vi "test Subset.vi"(8 "error in (no error)":errorcluster, 11 "TestCase in":refnum<class "Buffers Tests.lvclass">) -> (0 "error out":errorcluster, 3 "TestCase out":refnum<class "Buffers Tests.lvclass">)   [LabVIEW 2017, in "Buffers Tests.lvclass"]
uses:
  Buffers Tests.lvclass
  Buffers Tests.lvclass/Buffers Tests.ctl
  Classes/Buffers/Buffers.lvclass/Buffers.ctl
  <vilib>/NI/Memory Manager/Classes/Pointer/Pointer.lvclass/Pointer.ctl
  <vilib>/NI/Memory Manager/Classes/Pointer/Get Address.vi
  <vilib>/NI/Memory Manager/Classes/Pointer/Get Size.vi
  Classes/Buffer/Buffer.lvclass
  C:/Program Files (x86)/National Instruments/LabVIEW 2017/vi.lib/NI/Memory Manager/Classes/Pointer/Pointer.lvclass
  <vilib>/addons/_JKI Toolkits/VI Tester/TestCase.llb/TestCase.lvclass
  Classes/Buffers/Buffers.lvclass
  C:/Program Files (x86)/National Instruments/LabVIEW 2017/vi.lib/addons/_JKI Toolkits/VI Tester/TestCase.llb/TestCase.lvclass
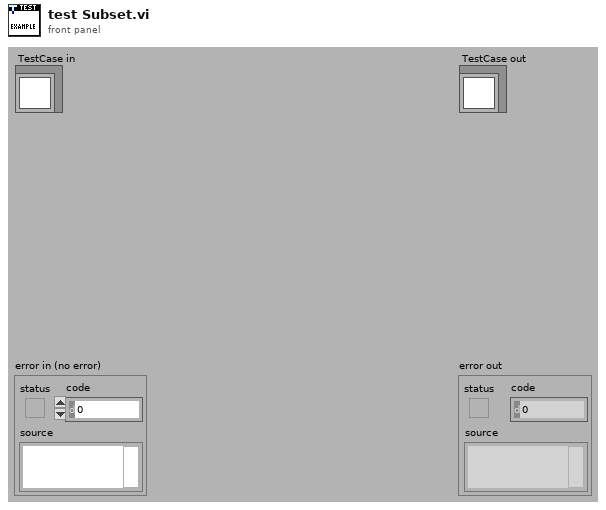
[diagram p1: front panel]
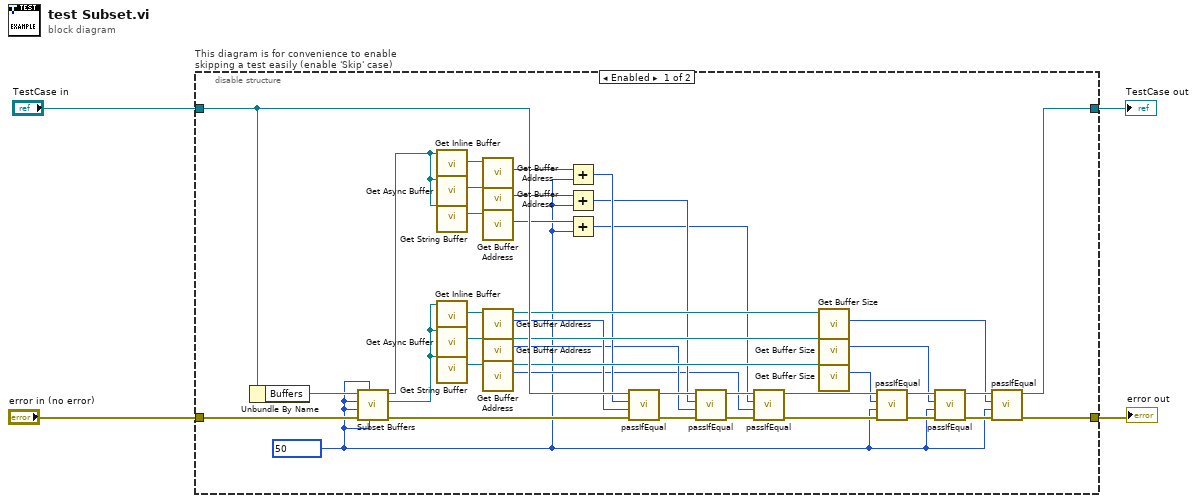
[diagram p0: block diagram]
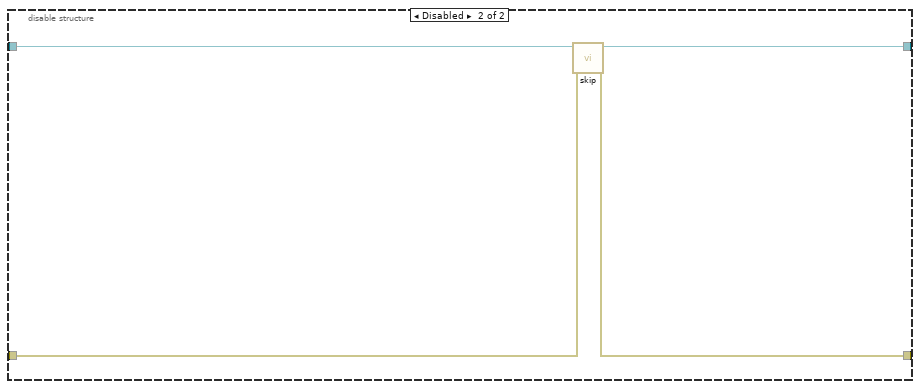
[diagram p2: hidden frame]
diagram:
  n1 = disable-structure "This diagram is for convenience to enable skipping a test easily (enable 'Skip' case)" shown="Enabled" {
    disable-tunnel: "TestCase in" -> [w44 w48]
    disable-tunnel: [w43 w46] -> w1
    disable-tunnel: [w42 w47] -> w3
    disable-tunnel: "error in (no error)" -> [w41 w45]
    frame Enabled {
      w9 = u64 50 ("string buffer size")
      n2 = Unbundle By Name(w44) -> ("Buffers"=w40:refnum<class "Buffers.lvclass">)
      n3 = call "Subset Buffers.vi"("inline buffer offset"=w9, "string buffer offset"=w9, "error in (no error)"=w41, "inline buffer size"=w9, "string buffer size"=w9, "Buffers in"=w40) -> ("error out"=w29:errorcluster, "subset Buffers"=w33:refnum<class "Buffers.lvclass">, "Buffers out"=w5:refnum<class "Buffers.lvclass">)  [unwired: 1 in, 2 out]
      n4 = call "Get Inline Buffer.vi"("Buffers in"=w5) -> ("Inline Buffer"=w39:refnum<class "Buffer.lvclass">)  [unwired: 9 in, 1 out]
      n5 = call "Get Async Buffer.vi"("Buffers in"=w5) -> ("Async Buffer"=w37:refnum<class "Buffer.lvclass">)  [unwired: 9 in, 1 out]
      n6 = call "Get String Buffer.vi"("Buffers in"=w5) -> ("String Buffer"=w38:refnum<class "Buffer.lvclass">)  [unwired: 9 in, 1 out]
      n7 = call "Get Inline Buffer.vi"("Buffers in"=w33) -> ("Inline Buffer"=w36:refnum<class "Buffer.lvclass">)  [unwired: 9 in, 1 out]
      n8 = call "Get Async Buffer.vi"("Buffers in"=w33) -> ("Async Buffer"=w34:refnum<class "Buffer.lvclass">)  [unwired: 9 in, 1 out]
      n9 = call "Get String Buffer.vi"("Buffers in"=w33) -> ("String Buffer"=w35:refnum<class "Buffer.lvclass">)  [unwired: 9 in, 1 out]
      n10 = call "Get Buffer Address.vi"("Buffer in"=w39) -> ("buffer address"=w28:u64)  [unwired: 9 in, 1 out]
      n11 = call "Get Buffer Address.vi"("Buffer in"=w37) -> ("buffer address"=w27:u64)  [unwired: 9 in, 1 out]
      n12 = call "Get Buffer Address.vi"("Buffer in"=w38) -> ("buffer address"=w26:u64)  [unwired: 9 in, 1 out]
      n13 = call "Get Buffer Address.vi"("Buffer in"=w36) -> ("buffer address"=w19:u64, "Buffer out"=w30:refnum<class "Buffer.lvclass">)  [unwired: 9 in]
      n14 = call "Get Buffer Address.vi"("Buffer in"=w34) -> ("buffer address"=w11:u64, "Buffer out"=w31:refnum<class "Buffer.lvclass">)  [unwired: 9 in]
      n15 = call "Get Buffer Address.vi"("Buffer in"=w35) -> ("buffer address"=w10:u64, "Buffer out"=w32:refnum<class "Buffer.lvclass">)  [unwired: 9 in]
      n16 = Add(x=w28, y=w9) -> (x+y=w25:u64)
      n17 = Add(x=w27, y=w9) -> (x+y=w13:u64)
      n18 = Add(x=w26, y=w9) -> (x+y=w12:u64)
      n19 = call-dynamic "passIfEqual.vi"("error in (no error)"=w29, "y"=w19, "x"=w25, "TestCase in"=w44) -> ("error out"=w24:errorcluster, "TestCase out"=w18:refnum<class "Buffers Tests.lvclass">)  [unwired: 6 in]
      n20 = call-dynamic "passIfEqual.vi"("error in (no error)"=w24, "y"=w11, "x"=w13, "TestCase in"=w18) -> ("error out"=w23:errorcluster, "TestCase out"=w17:refnum<class "Buffers Tests.lvclass">)  [unwired: 6 in]
      n21 = call-dynamic "passIfEqual.vi"("error in (no error)"=w23, "y"=w10, "x"=w12, "TestCase in"=w17) -> ("error out"=w22:errorcluster, "TestCase out"=w16:refnum<class "Buffers Tests.lvclass">)  [unwired: 6 in]
      n22 = call "Get Buffer Size.vi"("Buffer in"=w30) -> ("buffer size"=w6:u64)  [unwired: 9 in, 1 out]
      n23 = call "Get Buffer Size.vi"("Buffer in"=w31) -> ("buffer size"=w7:u64)  [unwired: 9 in, 1 out]
      n24 = call "Get Buffer Size.vi"("Buffer in"=w32) -> ("buffer size"=w8:u64)  [unwired: 9 in, 1 out]
      n25 = call-dynamic "passIfEqual.vi"("error in (no error)"=w22, "y"=w9, "x"=w8, "TestCase in"=w16) -> ("error out"=w21:errorcluster, "TestCase out"=w15:refnum<class "Buffers Tests.lvclass">)  [unwired: 6 in]
      n26 = call-dynamic "passIfEqual.vi"("error in (no error)"=w21, "y"=w9, "x"=w7, "TestCase in"=w15) -> ("error out"=w20:errorcluster, "TestCase out"=w14:refnum<class "Buffers Tests.lvclass">)  [unwired: 6 in]
      n27 = call-dynamic "passIfEqual.vi"("error in (no error)"=w20, "y"=w9, "x"=w6, "TestCase in"=w14) -> ("error out"=w42:errorcluster, "TestCase out"=w43:refnum<class "Buffers Tests.lvclass">)  [unwired: 6 in]
    }
    frame Disabled {
      # "skip test result while test is under development"
      n28 = call <vilib>:"skip.vi"("error in (no error)"=w45, "TestCase in"=w48) -> ("error out"=w47:errorcluster, "TestCase out"=w46:refnum<class "Buffers Tests.lvclass">)  [unwired: 8 in]
    }
  }
  "error out" <- w3
  "TestCase out" <- w1
